vi "Acq_askComents.vi"(4 "Folder path":path=path "C:/VIP Module x2/Files/Acquisition/yyyymmdd_hh-mm-ss") -> (1 "Complete file path":path=path "C:/VIP Module x2/Files/Acquisition/yyyymmdd_hh-mm-ss")   [LabVIEW 2015, in "VIPM2.lvlib"]
doc: "In a new windows, ask user to edit a comment to attach inside the file name."
uses:
  VIPM2.lvlib
panel:
  out "rest chars":i32=144 caption="Chars to limit"
  in  "Validate Button":bool
  in  "Comments":string="Acquisition_DATA"
  # "Optionally, write comments within the file name"
  # "Do not use these characters:    \\  /  :  *  ?  \"  <  >  |"
  # "To keep file integrity, comments are limited to 160 chars"
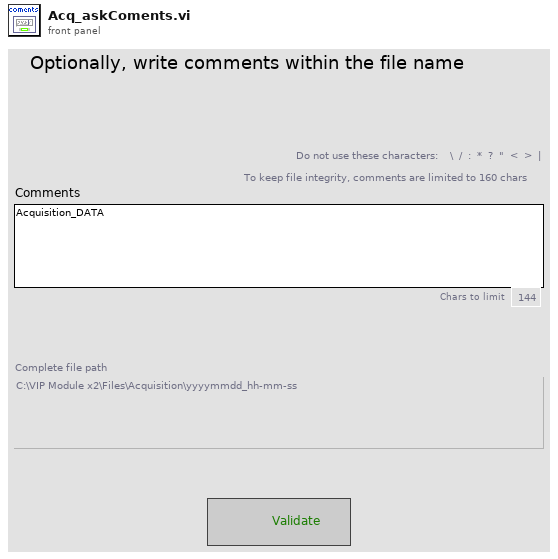
[diagram p1: front panel]
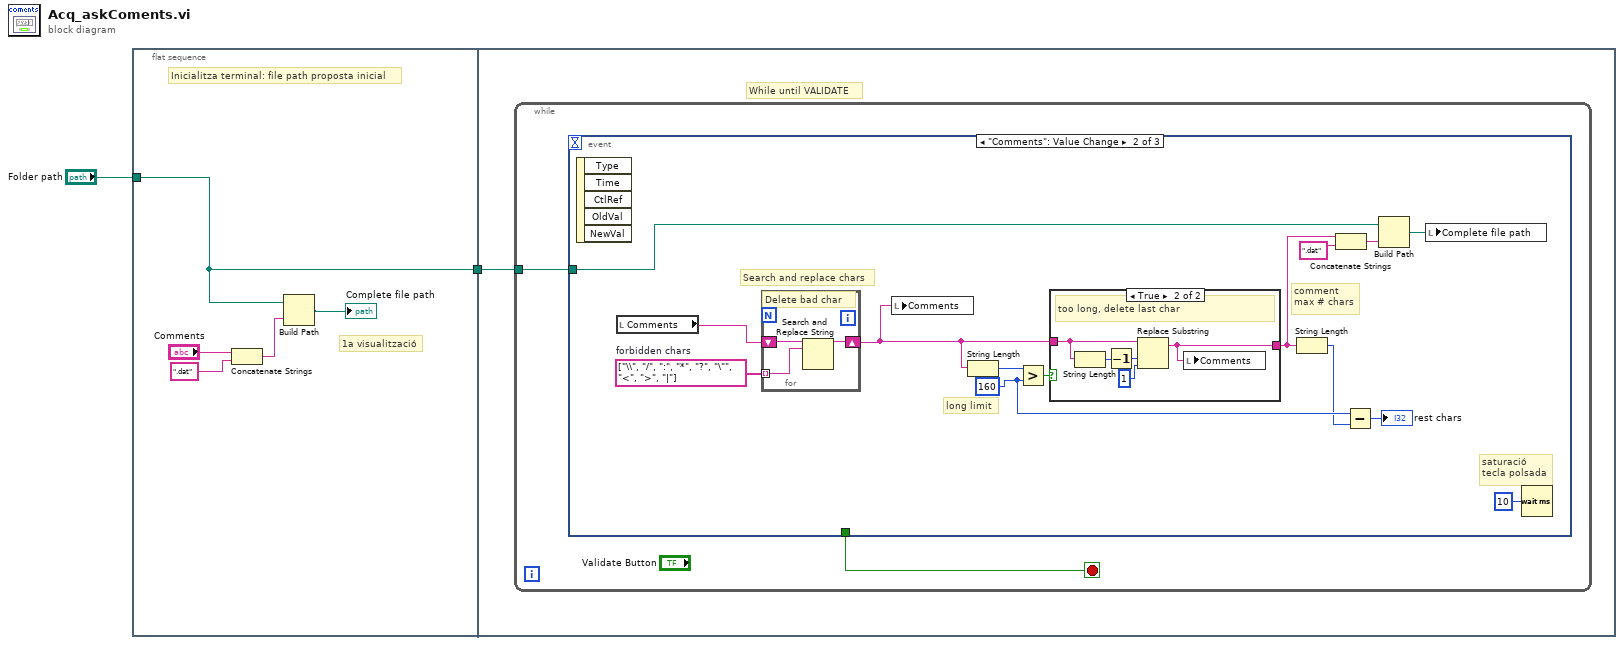
[diagram p0: block diagram]
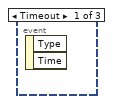
[diagram p2: hidden frame]
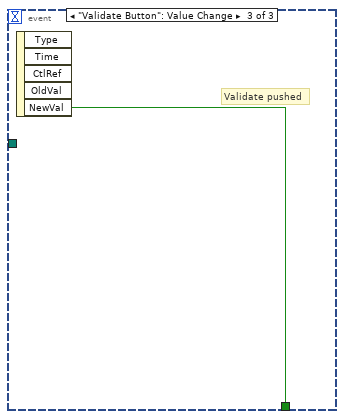
[diagram p4: hidden frame]
diagram:
  n1 = flat-sequence {
    tunnel: "Folder path" -> [w4]
    tunnel: [w4] -> w1
    tunnel: w1 -> [w8]
    frame #0 {
      # "1a visualització"
      # "Inicialitza terminal: file path proposta inicial"
      n2 = Concatenate Strings "Concatenate Strings"("Comments", ".dat" ("string")) -> (w3:string)
      n3 = Build Path(base path=w4, name or relative path=w3) -> (appended path=→"Complete file path":path)
    }
    frame #1 {
      # "While until VALIDATE"
      n4 = while {
        tunnel: w8 -> [w10]
        stop <- w9 stop-if-true
        n5 = event shown="[1] \"Comments\": Value Change" {
          selector: _ -> [_ _ _]
          dyn-events: _ -> [_ _ _]
          timeout: _ -> [_ _ _]
          tunnel: w10 -> [_ w12 _]
          tunnel: [_ _ w34] -> w9
          event Timeout {
            n6 = event-data() -> ()  [unwired: 1 in, 2 out]
          }
          event "Comments": Value Change {
            w20 = 160 ("y")
            w24 = string[] ["\\", "/", ":", "*", "?", "\"", "<", ">", "|"]  # forbidden chars
            # "Search and replace chars"
            # "comment\nmax # chars"
            # "long limit"
            # "saturació\ntecla polsada"
            n7 = event-data() -> ()  [unwired: 1 in, 5 out]
            n8 = local read "Comments"() -> (w15:string)
            n9 = for {
              tunnel: w24 -> [w32] mode=indexing
              shift-right: [w31] -> w14
              shift-left: w15 -> [w33]
              # "Delete bad char"
              n10 = Search and Replace String(input string=w33, search string=w32) -> (result string=w31:string)  [unwired: 6 in, 3 out]
            }
            n11 = local write "Comments"(w14) -> ()
            n12 = String Length(string=w14) -> (length=w19:i32)
            n13 = Greater?(x=w19, y=w20) -> (0:w21:bool)
            n14 = case shown="True" w21 {
              tunnel: w14 -> [w25 w27]
              tunnel: [w25 w26] -> w17
              frame False {
                # "long <= limit     OK"
              }
              frame True {
                # "too long, delete last char"
                n15 = String Length(string=w27) -> (length=w30:i32)
                n16 = Decrement(x=w30) -> (x-1=w29:i32)
                n17 = Replace Substring(2:1 ("length (len. of substring)"), 3:w29, 5:w27) -> (1:w26:string)  [unwired: 1 in, 1 out]
                n18 = local write "Comments"(w26) -> ()
              }
            }
            n19 = String Length(string=w17) -> (length=w16:i32)
            n20 = Concatenate Strings "Concatenate Strings"(w17, ".dat" ("string")) -> (w13:string)
            n21 = Subtract(x=w20, y=w16) -> (x-y=→"rest chars":i32)
            n22 = Build Path(base path=w12, name or relative path=w13) -> (appended path=w11:path)
            n23 = local write "Complete file path"(w11) -> ()
            n24 = Wait (ms)(milliseconds to wait=u32 10) -> ()  [unwired: 1 out]
          }
          event "Validate Button": Value Change {
            # "Validate pushed"
            n25 = event-data() -> ("NewVal"=w34:bool)  [unwired: 1 in, 4 out]
          }
        }
      }
    }
  }
